vi "AdvBGSub.vi"(8 "error in":errorcluster, 11 "Refnum in":T2) -> (0 "error out":errorcluster, 2 "-x":sgl, 3 "Refnum out":T2, 4 "empty image":bool)   [LabVIEW 2020]
uses:
  IMAQ Image.ctl
  NI_Vision_Development_Module.lvlib
panel:
  out "Histogram Report":T1 {"Standard  Variation" format="%.2f"; "Mean Value" format="%.2f"; "Interval Width" format="%.2f"; "Starting Value" format="%.2f"; "Maximal Value" format="%.2f"; "Minimal Value" format="%.2f"}
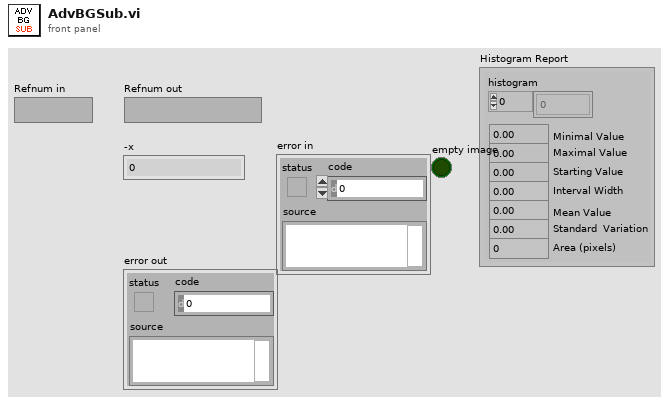
[diagram p1: front panel]
types:
  T1 = cluster{"histogram":u32[], "Minimal Value":sgl, "Maximal Value":sgl, "Starting Value":sgl, "Interval Width":sgl, "Mean Value":sgl, "Standard  Variation":sgl, "Area (pixels)":i32}
  T2 = typedef "IMAQ Image.ctl" = refnum<image>
  T3 = typedef "Image Type" = u32
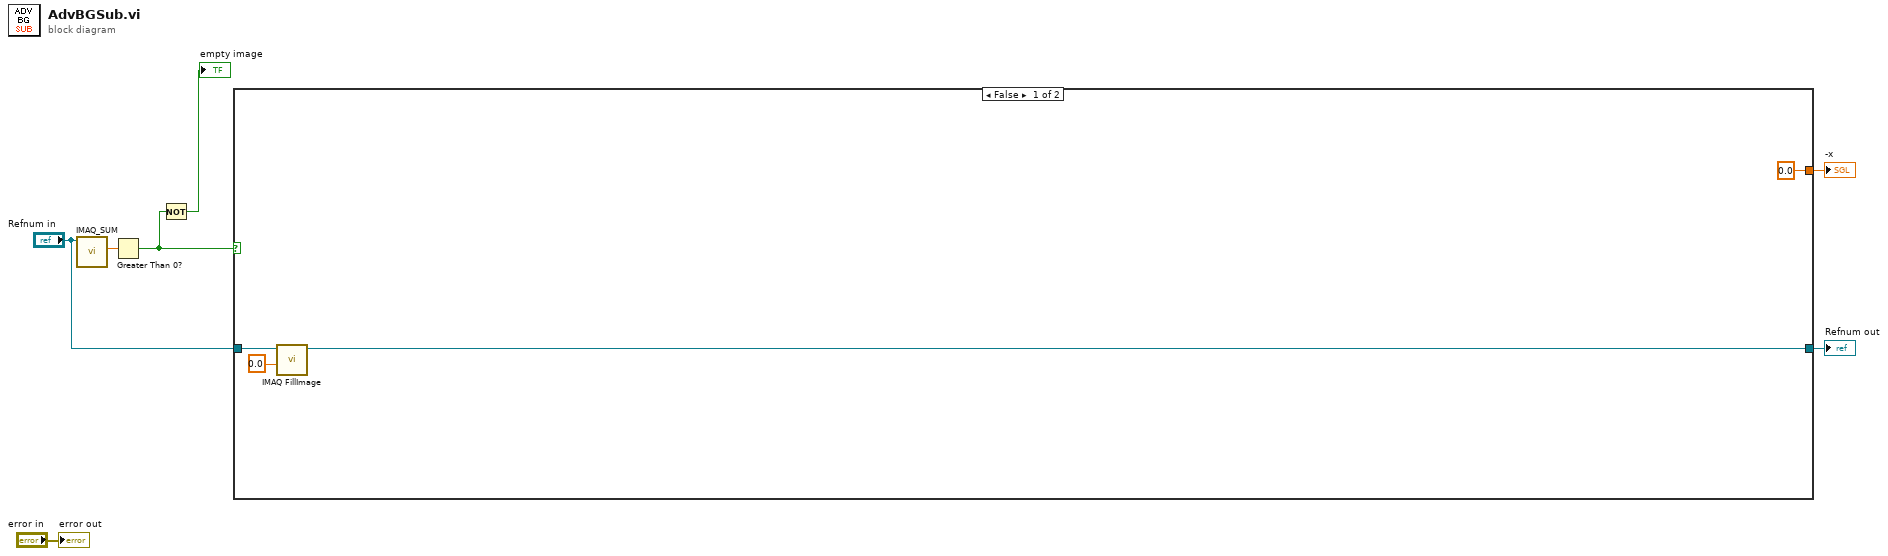
[diagram p0: block diagram]
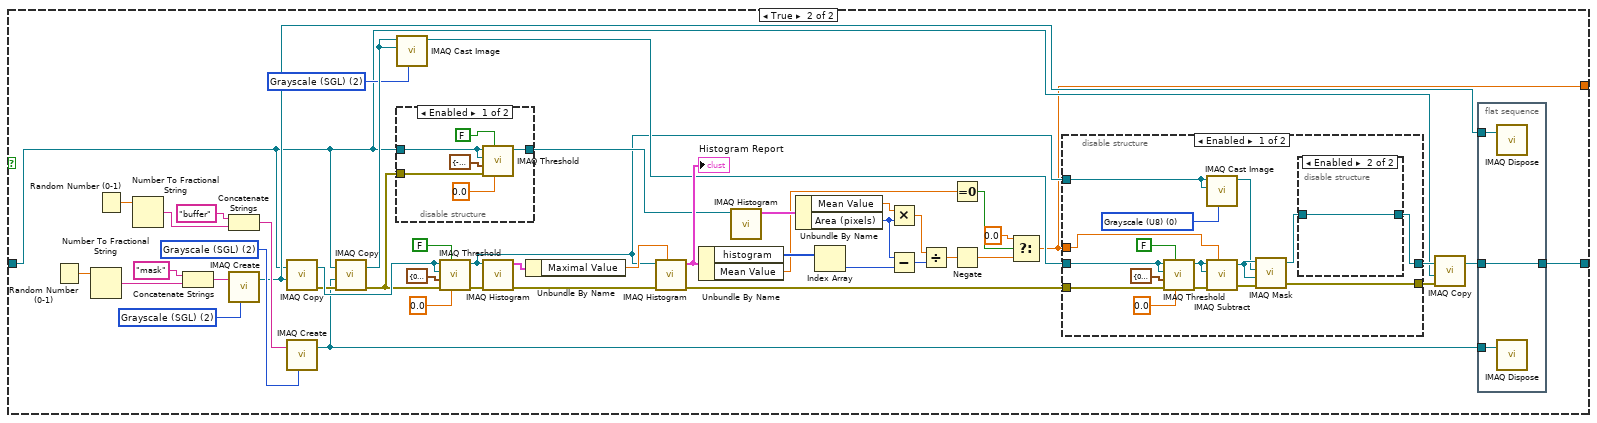
[diagram p2: hidden frame]
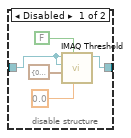
[diagram p4: hidden frame]
diagram:
  n1 = call "IMAQ_SUM.vi"("Image"="Refnum in") -> ("Sum"=w3:sgl)  [unwired: 9 in, 1 out]
  n2 = Greater Than 0?(x=w3) -> (x > 0?=w2:bool)
  n3 = Not(x=w2) -> (.not. x?=→"empty image":bool)
  n4 = case shown="False" w2 {
    tunnel: "Refnum in" -> [w9 w22]
    tunnel: [w8 w21] -> w5
    tunnel: [sgl 0.0 w19] -> w4
    frame False {
      n5 = call "IMAQ FillImage"("Pixel Value (U8, U16, I16, Float)"=sgl 0.0, "Image"=w9) -> ("Image Out"=w8:T2)  [unwired: 8 in, 1 out]
    }
    frame True {
      w31 = T3 2 items=["Grayscale (U8)", "Grayscale (I16)", "Grayscale (SGL)", "Complex (CSG)", "RGB (U32)", "HSL (U32)", "RGB (U64)", "Grayscale (U16)"] ("Image Type")
      w36 = T3 2 items=["Grayscale (U8)", "Grayscale (I16)", "Grayscale (SGL)", "Complex (CSG)", "RGB (U32)", "HSL (U32)", "RGB (U64)", "Grayscale (U16)"] ("Image Type")
      w56 = T3 2 items=["Grayscale (U8)", "Grayscale (I16)", "Grayscale (SGL)", "Complex (CSG)", "RGB (U32)", "HSL (U32)", "RGB (U64)", "Grayscale (U16)"] ("Image Type")
      n6 = Random Number (0-1)() -> (number: 0 to 1=w38:dbl)
      n7 = Number To Fractional String(number=w38) -> (F-format string=w40:string)  [unwired: 3 in]
      n8 = Random Number (0-1)() -> (number: 0 to 1=w34:dbl)
      n9 = Number To Fractional String(number=w34) -> (F-format string=w32:string)  [unwired: 3 in]
      n10 = Concatenate Strings("mask" ("Image Name"), w40) -> (w37:string)
      n11 = Concatenate Strings("buffer" ("Image Name"), w32) -> (w35:string)
      n12 = call "IMAQ Create"("Image Name"=w37, "Image Type"=w36) -> ("New Image"=w30:T2)  [unwired: 3 in, 1 out]
      n13 = call "IMAQ Copy"("Image Dst"=w30, "Image Src"=w22) -> ("error out"=w15:errorcluster, "Image Dst Out"=w52:T2)  [unwired: 4 in]
      n14 = call "IMAQ Create"("Image Name"=w35, "Image Type"=w31) -> ("New Image"=w12:T2)  [unwired: 3 in, 1 out]
      n15 = call "IMAQ Copy"("error in (no error)"=w15, "Image Dst"=w12, "Image Src"=w22) -> ("error out"=w14:errorcluster, "Image Dst Out"=w57:T2)  [unwired: 3 in]
      n16 = call "IMAQ Cast Image"("Image Type"=w56, "Image Dst"=w57, "Image Src"=w57) -> ("Image Dst Out"=w29:T2)  [unwired: 7 in, 1 out]
      n17 = disable-structure shown="Enabled" {
        disable-tunnel: [w64 w68] -> w43
        disable-tunnel: w22 -> [w63 w68]
        disable-tunnel: w14 -> [w62 _]
        frame Enabled {
          n18 = call "IMAQ Threshold"("Replace Value"=sgl 0.0, "Keep/Replace Value (Replace)"=FALSE, "error in (no error)"=w62, "Range"=cluster{"Lower value":sgl, "Upper value":sgl} {"Lower value"=-99999.0, "Upper value"=0.0}, "Image Dst"=w63, "Image Src"=w63) -> ("Image Dst Out"=w64:T2)  [unwired: 4 in, 1 out]
        }
        frame Disabled {
        }
      }
      n19 = call "IMAQ Threshold"("Replace Value"=sgl 0.0, "Keep/Replace Value (Replace)"=FALSE, "error in (no error)"=w14, "Range"=cluster{"Lower value":sgl, "Upper value":sgl} {"Lower value"=0.0, "Upper value"=99999.0}, "Image Dst"=w52, "Image Src"=w52) -> ("error out"=w16:errorcluster, "Image Dst Out"=w26:T2)  [unwired: 4 in]
      n20 = call "IMAQ Histogram"("error in (no error)"=w16, "Image"=w26) -> ("error out"=w13:errorcluster, "Histogram Report"=w51:T1)  [unwired: 8 in]
      n21 = Unbundle By Name(w51) -> ("Maximal Value"=w45:sgl)
      n22 = call "IMAQ Histogram"("Number of Classes"=w45, "error in (no error)"=w13, "Image"=w26) -> ("error out"=w17:errorcluster, "Histogram Report"=w49:T1)  [unwired: 7 in]
      "Histogram Report" <- w49
      n23 = Unbundle By Name(w49) -> ("histogram"=w48:u32[], "Mean Value"=w25:sgl)
      n24 = call "IMAQ Histogram"("Image"=w43) -> ("Histogram Report"=w50:T1)  [unwired: 9 in, 1 out]
      n25 = Unbundle By Name(w50) -> ("Mean Value"=w44:sgl, "Area (pixels)"=w41:i32)
      n26 = Index Array(array=w48) -> (element=w47:u32)  [unwired: 1 in]
      n27 = Multiply(x=w44, y=w41) -> (x*y=w42:sgl)
      n28 = Subtract(x=w41, y=w47) -> (x-y=w46:u32)
      n29 = Divide(x=w42, y=w46) -> (x/y=w58:sgl)
      n30 = Equal To 0?(x=w25) -> (x = 0?=w24:bool)
      n31 = Negate(x=w58) -> (-x=w20:sgl)
      n32 = Select(t=0.0, s=w24, f=w20) -> (s? t:f=w19:dbl)
      n33 = disable-structure shown="Enabled" {
        disable-tunnel: w19 -> [w84 _]
        disable-tunnel: [w83 w91] -> w28
        disable-tunnel: w29 -> [w80 w91]
        disable-tunnel: w26 -> [w74 _]
        disable-tunnel: [w71 _] -> w18
        disable-tunnel: w17 -> [w69 _]
        frame Enabled {
          w73 = T3 0 items=["Grayscale (U8)", "Grayscale (I16)", "Grayscale (SGL)", "Complex (CSG)", "RGB (U32)", "HSL (U32)", "RGB (U64)", "Grayscale (U16)"] ("Image Type")
          n34 = call "IMAQ Threshold"("Replace Value"=sgl 0.0, "Keep/Replace Value (Replace)"=FALSE, "error in (no error)"=w69, "Range"=cluster{"Lower value":sgl, "Upper value":sgl} {"Lower value"=0.0, "Upper value"=9999999.0}, "Image Dst"=w80, "Image Src"=w80) -> ("error out"=w70:errorcluster, "Image Dst Out"=w78:T2)  [unwired: 4 in]
          n35 = call "IMAQ Cast Image"("Image Type"=w73, "Image Dst"=w74, "Image Src"=w74) -> ("Image Dst Out"=w72:T2)  [unwired: 7 in, 1 out]
          n36 = call "IMAQ Subtract"("Image Src A"=w78, "Constant"=w84, "Image Dst"=w78, "error in (no error)"=w70) -> ("Image Dst Out"=w76:T2, "error out"=w77:errorcluster)  [unwired: 3 in]
          n37 = call "IMAQ Mask"("error in (no error)"=w77, "Image Dst"=w76, "Image Mask"=w72, "Image Src"=w76) -> ("error out"=w71:errorcluster, "Image Dst Out"=w75:T2)  [unwired: 1 in]
          n38 = disable-structure shown="Enabled" {
            disable-tunnel: [w86 w90] -> w83
            disable-tunnel: w75 -> [w85 w90]
            frame Disabled {
              n39 = call "IMAQ Threshold"("Replace Value"=sgl 0.0, "Keep/Replace Value (Replace)"=FALSE, "Range"=cluster{"Lower value":sgl, "Upper value":sgl} {"Lower value"=0.0, "Upper value"=9999999.0}, "Image Dst"=w85, "Image Src"=w85) -> ("Image Dst Out"=w86:T2)  [unwired: 5 in, 1 out]
            }
            frame Enabled {
            }
          }
        }
        frame Disabled {
        }
      }
      n40 = call "IMAQ Copy"("error in (no error)"=w18, "Image Dst"=w22, "Image Src"=w28) -> ("Image Dst Out"=w27:T2)  [unwired: 3 in, 1 out]
      n41 = flat-sequence {
        tunnel: w27 -> [w60]
        tunnel: w30 -> [w61]
        tunnel: [w60] -> w21
        tunnel: w12 -> [w59]
        frame #0 {
          n42 = call "IMAQ Dispose"("Image"=w61) -> ()  [unwired: 5 in, 1 out]
          n43 = call "IMAQ Dispose"("Image"=w59) -> ()  [unwired: 5 in, 1 out]
        }
      }
    }
  }
  "Refnum out" <- w5
  "-x" <- w4
  "error out" <- "error in"
